vi "Control - Generic - Direct Injection Host.vi"() -> ()   [LabVIEW 2015, in "ECS-Host.lvlib"]
uses:
  ECS-Host.lvlib
  <vilib>/addons/Software Calibration Management/XControls/TBL2D.xctl
  <vilib>/addons/Software Calibration Management/XControls/TBL1D.xctl
panel:
  in  "CylFuelSplit":sgl[](array[numeric]) caption="[%]" format="%#_3g"
  out "InjQty_Calc":sgl[](array[numeric]) caption="[mg/cyc/cyl]" format="%_4g"
  out "_Cylinder ID":string[](array[string])
  out "MainSOIAdv_TblOut":sgl caption="[CAD]" format="%#.3g"
  in  "MainSOIAdv_Tbl":cluster{"X":sgl[], "Y":sgl[]}(xcontrol)
  in  "NxtCycQty_E":bool caption="Next Cycle DI Quantity Enable"
  in  "NxtCycSOI_E":bool caption="Next Cycle DI Timing Enable"
  out "AvgNextCycleOutput":sgl caption="[]" format="%#.3g"
  in  "Pilot1SOI_ManE":bool
  in  "Post2SOI_Man":sgl caption="[]"
  in  "Post1SOI_Man":sgl caption="[]"
  in  "MainSOI_Man":sgl caption="[]"
  in  "Pilot2SOI_Man":sgl caption="[]"
  in  "Pilot1SOI_Man":sgl caption="[DBTDC]"
  in  "Post2SOI_ManE":bool
  in  "Post1SOI_ManE":bool
  in  "MainSOI_ManE":bool
  in  "Pilot2SOI_ManE":bool
  out "Post2SOI_TblOut":sgl caption="[]" format="%#.3g"
  out "Post1SOI_TblOut":sgl caption="[]" format="%#.3g"
  out "MainSOI_TblOut":sgl caption="[]" format="%#.3g"
  out "Pilot2SOI_TblOut":sgl caption="[]" format="%#.3g"
  out "Pilot1SOI_TblOut":sgl caption="[DBTDC]" format="%#.3g"
  in  "_SOI Table":T1(tab)=enum."Main" caption="Fuel Injection Timing Tables"
  in  "Pilot1SOI_Tbl":cluster{"X":sgl[], "Y":sgl[], "Z":sgl[][]}(xcontrol) caption="[]"
  in  "Pilot2SOI_Tbl":cluster{"X":sgl[], "Y":sgl[], "Z":sgl[][]}(xcontrol) caption="[]"
  in  "MainSOI_Tbl":cluster{"X":sgl[], "Y":sgl[], "Z":sgl[][]}(xcontrol) caption="[]"
  in  "Post1SOI_Tbl":cluster{"X":sgl[], "Y":sgl[], "Z":sgl[][]}(xcontrol) caption="[]"
  in  "Post2SOI_Tbl":cluster{"X":sgl[], "Y":sgl[], "Z":sgl[][]}(xcontrol) caption="[]"
  in  "Pilot1Qty_ManE":bool
  in  "Post2Qty_Man":sgl caption="[]"
  in  "Post1Qty_Man":sgl caption="[]"
  in  "MainQty_Man":sgl caption="[]"
  in  "Pilot2Qty_Man":sgl caption="[]"
  in  "Pilot1Qty_Man":sgl caption="[mg/cyc]"
  in  "Post2Qty_ManE":bool
  in  "Post1Qty_ManE":bool
  in  "MainQty_ManE":bool
  in  "Pilot2Qty_ManE":bool
  out "Post2Split_TblOut":sgl caption="[]" format="%#.3g"
  out "Post1Split_TblOut":sgl caption="[]" format="%#.3g"
  out "MainSplit_TblOut":sgl caption="[]" format="%#.3g"
  out "Pilot2Split_TblOut":sgl caption="[]" format="%#.3g"
  out "Pilot1Split_TblOut":sgl caption="[%]" format="%#.3g"
  in  "_Quantity Table":T1(tab)=enum."Main" caption="Fuel Injection Split Tables"
  in  "Pilot1Split_Tbl":cluster{"X":sgl[], "Y":sgl[], "Z":sgl[][]}(xcontrol) caption="[]"
  in  "Pilot2Split_Tbl":cluster{"X":sgl[], "Y":sgl[], "Z":sgl[][]}(xcontrol) caption="[]"
  in  "MainSplit_Tbl":cluster{"X":sgl[], "Y":sgl[], "Z":sgl[][]}(xcontrol) caption="[]"
  in  "Post1Split_Tbl":cluster{"X":sgl[], "Y":sgl[], "Z":sgl[][]}(xcontrol) caption="[]"
  in  "Post2Split_Tbl":cluster{"X":sgl[], "Y":sgl[], "Z":sgl[][]}(xcontrol) caption="[]"
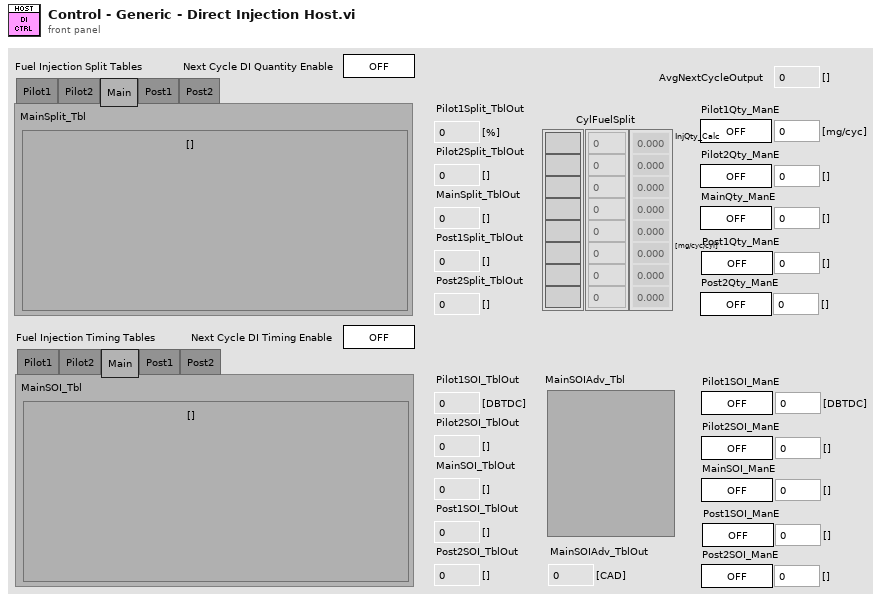
[diagram p1: front panel]
types:
  T1 = enum32{"Pilot1", "Pilot2", "Main", "Post1", "Post2"}
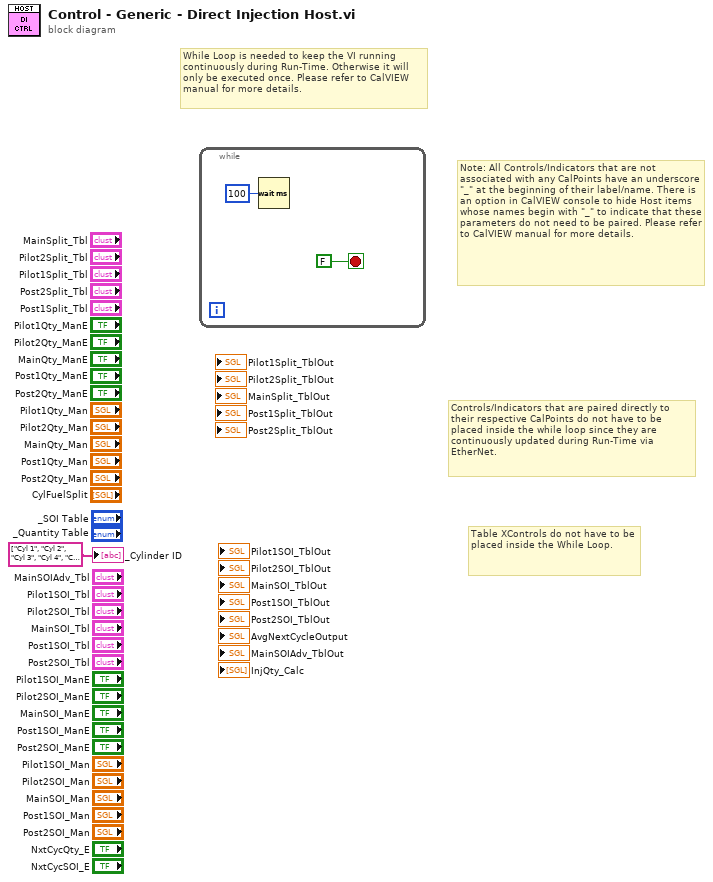
[diagram p0: block diagram]
diagram:
  # "Controls/Indicators that are paired directly to their respective CalPoints do not have to be placed inside the while loop since they are continuously updated during Run-Time via EtherNet."
  # "Table XControls do not have to be placed inside the While Loop."
  # "While Loop is needed to keep the VI running\ncontinuously during Run-Time. Otherwise it will only be executed once. Please refer to CalVIEW manual for more details."
  # "Note: All Controls/Indicators that are not associated with any CalPoints have an underscore \"_\" at the beginning of their label/name. There is an option in CalVIEW console to hide Host items whose names begin with \"_\" to indicate that these parameters do not need to be paired. Please refer to CalVIEW manual for more details."
  n1 = while {
    stop <- FALSE stop-if-true
    n2 = Wait (ms)(milliseconds to wait=u32 100) -> ()  [unwired: 1 out]
  }
  "_Cylinder ID" <- string[] ["Cyl 1", "Cyl 2", "Cyl 3", "Cyl 4", "Cyl 5", "Cyl 6", "Cyl 7", "Cyl 8"] ("_Cylinder ID")
